vi "Merc_Connection_Check.vi"(0 "VISA resource name":refnum<visa-resource-name>="GPIB0::24::1::INSTR", 1 "IP Address":string, 5 "Comms Layer":T1=enum."GPIB", 7 "Serial Configuration":T3={"Baud Rate"=9600, "Parity"=0, "Data Bits"=8, "Stop Bits"=20, "Flow Control"=0} {"Flow Control" items=["None", "XON/XOFF", "RTS/CTS", "XON/XOFF & RTS/CTS", "DTR/DSR", "XON/XOFF & DTR/DSR"]; "Stop Bits" items=["1.0"=10, "2.0"=20]; "Data Bits" items=["7"=7, "8"=8]; "Parity" items=["None", "Odd", "Even"]; "Baud Rate" items=["300"=300, "600"=600, "1200"=1200, "2400"=2400, "4800"=4800, "9600"=9600, "19200"=19200]}, 9 "ID Query (True)":bool, 12 "Clear Previous Connections (False)":bool, 13 "ISOBUS address":T2=-1 caption="ISOBUS address (-1)") -> (3 "Installed Devices":string[](array[string]), 14 "Valid?":T4, 15 "error out":errorcluster)   [LabVIEW 2013]
uses:
  <instrlib>/Mercury iXX/Public/Controls/Comms Transport Layer.ctl
  <instrlib>/Mercury iXX/Public/Controls/Serial Settings.ctl
  <instrlib>/Mercury iXX/Public/Controls/ISOBus Address.ctl
  <instrlib>/Mercury iXX/Public/Controls/Is Valid LED.ctl
  <instrlib>/Mercury iXX/Public/Libraries/System/Open/Open System.vi
  <instrlib>/Mercury iXX/Public/Libraries/System/Read/Catalogue (Read).vi
  <instrlib>/Mercury iXX/Public/Libraries/System/Read/Date (Read).vi
  <instrlib>/Mercury iXX/Public/Libraries/System/Read/FVer (Read).vi
  <instrlib>/Mercury iXX/Public/Libraries/System/Read/Serial Number (Read).vi
  <instrlib>/Mercury iXX/Public/Libraries/System/Read/Time (Read).vi
  <instrlib>/Mercury iXX/Mercury iXX.lvlib
  <instrlib>/Mercury iXX/Public/Libraries/System.lvlib
panel:
  in  "stop":bool
  in  "Tab Control":enum32{"Connection", "Devices"}(tab)
  out "VISA Comms Layer Notes":string
  in  "Connect":bool
  out "Connected?":bool
  out "Firmware Version":string
  out "Main Board Serial Number":string
  out "Mercury Sys Date":string
  out "Mercury Sys Time":string
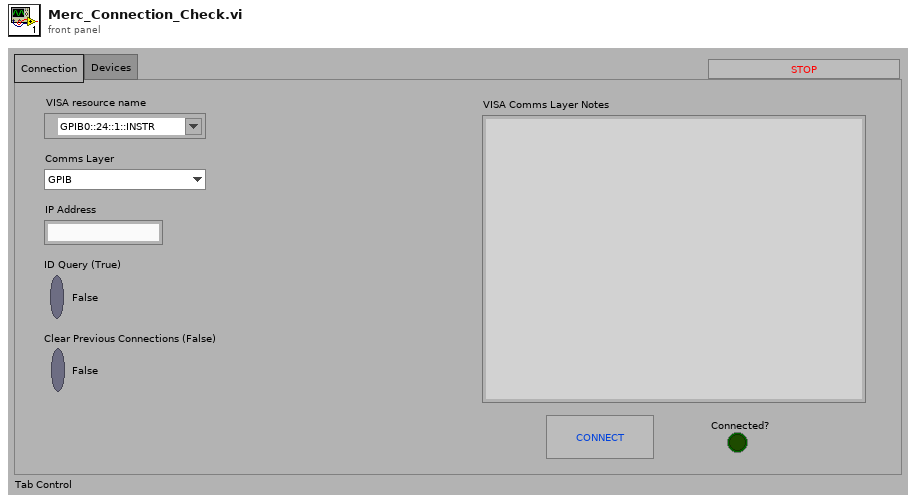
[diagram p1: front panel]
types:
  T1 = typedef "Mercury iXX.lvlib/Comms Transport Layer.ctl" = enum16{"Ethernet TCP/IP", "USB", "ISOBus - RS-232", "GPIB"}
  T2 = typedef "Mercury iXX.lvlib/ISOBus Address.ctl" = i32
  T3 = typedef "Mercury iXX.lvlib/Serial Settings.ctl" = cluster{"Baud Rate":u32, "Parity":u16, "Data Bits":u16, "Stop Bits":u16, "Flow Control":u16}
  T4 = typedef "Mercury iXX.lvlib/Is Valid LED.ctl" = bool
  T5 = typedef "Mercury iXX.lvlib/Mercury Reference.ctl" = cluster{"Comms":refnum<visa-resource-name>, "Device ID":string[], "Comms Layer":T1, "Command":string, "Query reference":T6}
  T6 = typedef "Mercury iXX.lvlib/Query Dynamic Reference.ctl" = refnum<vi>
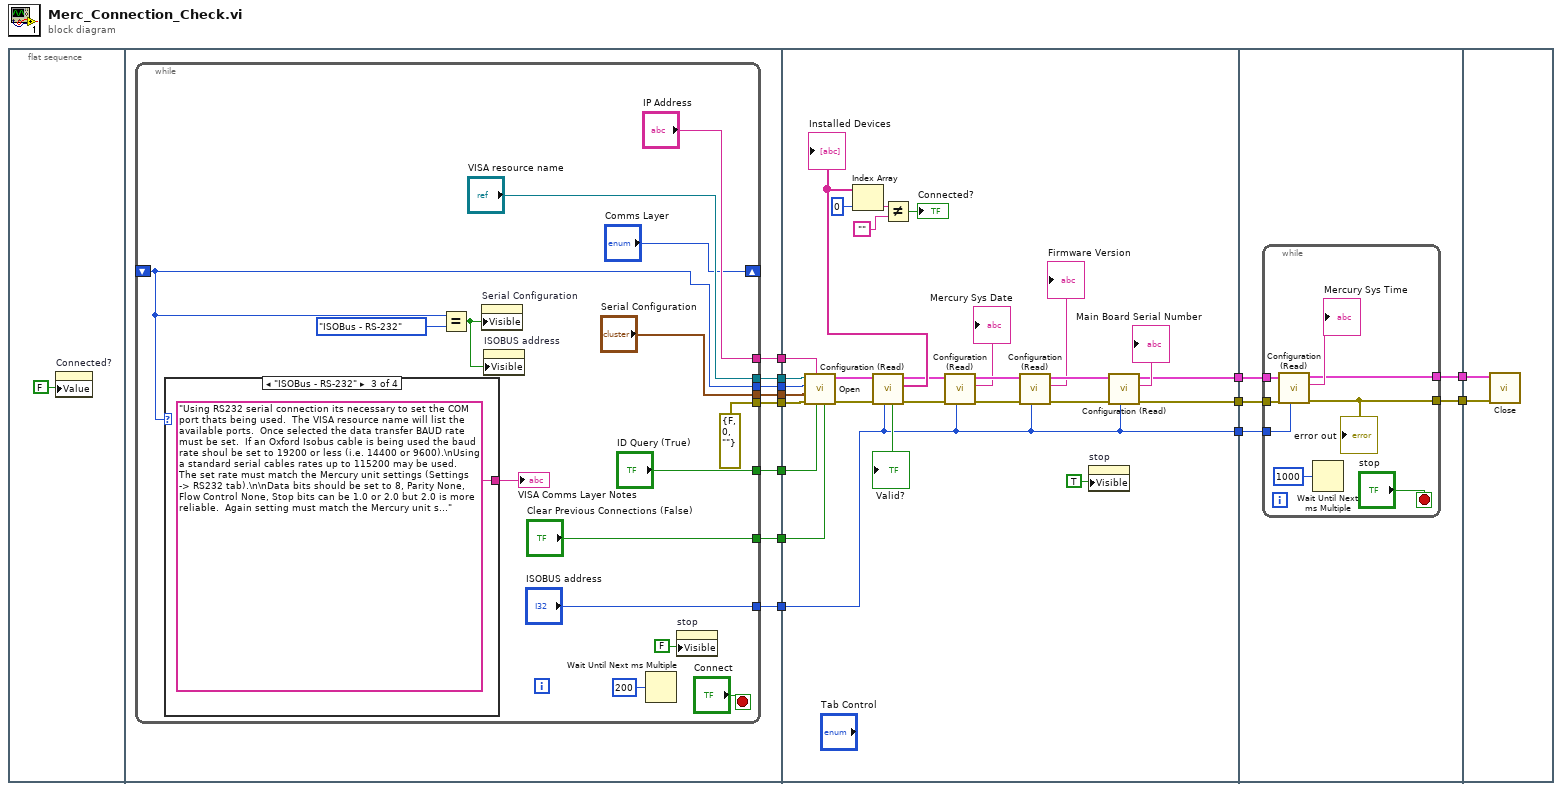
[diagram p0: block diagram]
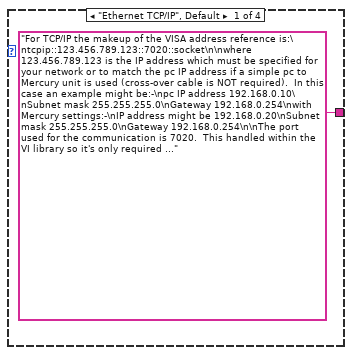
[diagram p2: hidden frame]
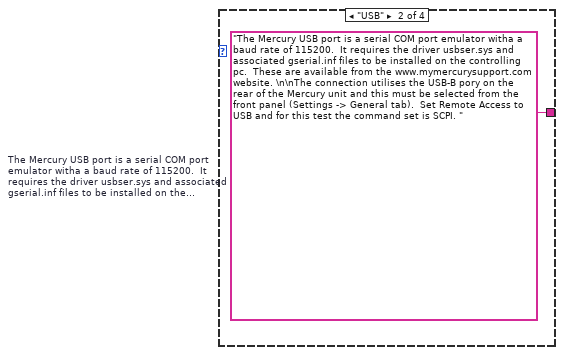
[diagram p3: hidden frame]
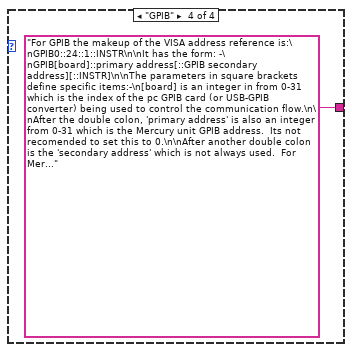
[diagram p4: hidden frame]
diagram:
  n1 = flat-sequence {
    tunnel: [w22] -> w13
    tunnel: [w21] -> w12
    tunnel: [w20] -> w11
    tunnel: [w19] -> w10
    tunnel: [w18] -> w9
    tunnel: [w17] -> w8
    tunnel: [w16] -> w7
    tunnel: [w15] -> w6
    tunnel: w13 -> [w64]
    tunnel: w12 -> [w63]
    tunnel: w11 -> [w65]
    tunnel: w10 -> [w66]
    tunnel: w9 -> [w67]
    tunnel: w8 -> [w69]
    tunnel: w7 -> [w68]
    tunnel: w6 -> [w43]
    tunnel: [w49] -> w5
    tunnel: [w43] -> w4
    tunnel: [w42] -> w3
    tunnel: w5 -> [w73]
    tunnel: w4 -> [w72]
    tunnel: w3 -> [w74]
    tunnel: [w71] -> w2
    tunnel: [w70] -> w1
    tunnel: w2 -> [w84]
    tunnel: w1 -> [w83]
    frame #0 {
      n2 = property on="Connected?" class="Bool (strict)"("Value"=FALSE ("x != y?")) -> ()  [unwired: 2 in, 2 out]
    }
    frame #1 {
      n3 = while {
        tunnel: ["VISA resource name"] -> w22
        tunnel: ["IP Address"] -> w21
        tunnel: [w25] -> w20
        tunnel: ["Serial Configuration"] -> w19
        tunnel: [errorcluster {"status"=FALSE, "code"=0, "source"=""} ("error in (no error)")] -> w18
        tunnel: ["ID Query (True)"] -> w17
        tunnel: ["Clear Previous Connections (False)"] -> w16
        tunnel: ["ISOBUS address"] -> w15
        shift-right: ["Comms Layer"] -> _
        shift-left: _ -> [w25]
        stop <- "Connect" stop-if-true
        n4 = case shown="\"ISOBus - RS-232\"" w25 {
          tunnel: ["For TCP/IP the makeup of the VISA address reference is:\ntcpip::123.456.789.123::7020::socket\n\nwhere 123.456.789.123 is the IP address which must be specified for your network or to match the pc IP address if a simple pc to Mercury unit is used (cross-over cable is NOT required).  In this case an example might be:-\npc IP address 192.168.0.10\nSubnet mask 255.255.255.0\nGateway 192.168.0.254\nwith Mercury settings:-\nIP address might be 192.168.0.20\nSubnet mask 255.255.255.0\nGateway 192.168.0.254\n\nThe port used for the communication is 7020.  This handled within the VI library so it's only required to set the IP address in the VI to Match the Mercury unit. \n\nTo use,TCP/IP must be selected from the Mercury front panel (Settings -> General tab).  Set Remote Access to Ethernet and for this test the command set is SCPI." w39 "Using RS232 serial connection its necessary to set the COM port thats being used.  The VISA resource name will list the available ports.  Once selected the data transfer BAUD rate must be set.  If an Oxford Isobus cable is being used the baud rate shoul be set to 19200 or less (i.e. 14400 or 9600).\nUsing a standard serial cables rates up to 115200 may be used.  The set rate must match the Mercury unit settings (Settings -> RS232 tab).\n\nData bits should be set to 8, Parity None, Flow Control None, Stop bits can be 1.0 or 2.0 but 2.0 is more reliable.  Again setting must match the Mercury unit settings.\n\nAlways set an Isobus address even if an Isobus cable is not used.  Some of the functions in the VI library expect an Isobus address when useing RS232 comms and will not respond if its missing.\n\nTo use, RS232 must be selected from the Mercury front panel (Settings -> General tab).  Set Remote Access to RS232 and for this test, the command set is SCPI." "For GPIB the makeup of the VISA address reference is:\nGPIB0::24::1::INSTR\n\nIt has the form: -\nGPIB[board]::primary address[::GPIB secondary address][::INSTR]\n\nThe parameters in square brackets define specific items:-\n[board] is an integer in from 0-31 which is the index of the pc GPIB card (or USB-GPIB converter) being used to control the communication flow.\n\nAfter the double colon, 'primary address' is also an integer from 0-31 which is the Mercury unit GPIB address.  Its not recomended to set this to 0.\n\nAfter another double colon is the 'secondary address' which is not always used.  For Mercury units it is used and set to 1.\n\nTo use, GPIB must be selected from the Mercury front panel (Settings -> General tab).  Set Remote Access to GPIB and for this test the command set is SCPI."] -> w28
          frame "Ethernet TCP/IP", Default {
          }
          frame "USB" {
            w39 = "The Mercury USB port is a serial COM port emulator witha a baud rate of 115200.  It requires the driver usbser.sys and associated gserial.inf files to be installed on the controlling pc.  These are available from the www.mymercurysupport.com website. \n\nThe connection utilises the USB-B pory on the rear of the Mercury unit and this must be selected from the front panel (Settings -> General tab).  Set Remote Access to USB and for this test the command set is SCPI. "  # The Mercury USB port is a serial COM port emulator witha a baud rate of 115200.  It requires the driver usbser.sys and associated gserial.inf files to be installed on the controlling pc.  These are available from the www.mymercurysupport.com website.   The connection utilises the USB-B pory on the rear of the Mercury unit and this must be selected from the front panel (Settings -> General tab).  Set Remote Access to USB and for this test the command set is SCPI.
          }
          frame "ISOBus - RS-232" {
          }
          frame "GPIB" {
          }
        }
        "VISA Comms Layer Notes" <- w28
        n5 = Equal?(x=w25, y=Comms_Transport_Layer."ISOBus - RS-232") -> (x = y?=w24:bool)
        n6 = property on="Serial Configuration" class="Clust (strict)"("Visible"=w24) -> ()  [unwired: 2 in, 2 out]
        n7 = property on="ISOBUS address" class="DigNum (strict)"("Visible"=w24) -> ()  [unwired: 2 in, 2 out]
        n8 = Wait Until Next ms Multiple(millisecond multiple=u32 200) -> ()  [unwired: 1 out]
        n9 = property on="stop" class="Bool"("Visible"=FALSE) -> ()  [unwired: 2 in, 2 out]
      }
    }
    frame #2 {
      n10 = call-poly <instrlib>:"Open.vi"("Clear Previous Connections (False)"=w68, "ID Query (True)"=w69, "IP Address"=w63, "error in (no error)"=w67, "Serial Configuration"=w66, "Comms Layer"=w65, "VISA resource name"=w64) -> ("error out"=w58:errorcluster, "Mercury Reference Out"=w59:T5)  [unwired: 3 out]
      n11 = call-poly <instrlib>:"Configuration (Read).vi"("ISOBUS address"=w43, "error in"=w58, "Mercury Reference In"=w59) -> ("error out"=w52:errorcluster, "Devices"=w56:string[], "Mercury Reference Out"=w53:T5, "Valid?"=→"Valid?":T4)  [unwired: 5 out]
      "Installed Devices" <- w56
      n12 = Index Array(array=w56, index=0) -> (element=w55:string)
      n13 = Not Equal?(x=w55, y="") -> (x != y?=→"Connected?":bool)
      n14 = call-poly <instrlib>:"Configuration (Read).vi"("ISOBUS address"=w43, "error in"=w52, "Mercury Reference In"=w53) -> ("error out"=w51:errorcluster, "Date"=→"Mercury Sys Date":string, "Mercury Reference Out"=w48:T5)  [unwired: 5 in, 1 out]
      n15 = call-poly <instrlib>:"Configuration (Read).vi"("ISOBUS address"=w43, "error in"=w51, "Mercury Reference In"=w48) -> ("error out"=w50:errorcluster, "Firmware Version"=→"Firmware Version":string, "Mercury Reference Out"=w47:T5)  [unwired: 5 in, 1 out]
      n16 = property on="stop" class="Bool"("Visible"=TRUE) -> ()  [unwired: 2 in, 2 out]
      n17 = call-poly <instrlib>:"Configuration (Read).vi"("ISOBUS address"=w43, "error in"=w50, "Mercury Reference In"=w47) -> ("error out"=w49:errorcluster, "Serial Number"=→"Main Board Serial Number":string, "Mercury Reference Out"=w42:T5)  [unwired: 5 in, 1 out]
    }
    frame #3 {
      n18 = while {
        tunnel: [w79] -> w71
        tunnel: [w78] -> w70
        tunnel: w74 -> [w77]
        tunnel: w73 -> [w76]
        tunnel: w72 -> [w75]
        stop <- "stop" stop-if-true
        n19 = call-poly <instrlib>:"Configuration (Read).vi"("ISOBUS address"=w75, "error in"=w76, "Mercury Reference In"=w77) -> ("error out"=w79:errorcluster, "Time"=→"Mercury Sys Time":string, "Mercury Reference Out"=w78:T5)  [unwired: 5 in, 1 out]
        "error out" <- w79
        n20 = Wait Until Next ms Multiple(millisecond multiple=u32 1000) -> ()  [unwired: 1 out]
      }
    }
    frame #4 {
      n21 = call <instrlib>:"Close.vi"("error in (no error)"=w84, "Mercury Reference"=w83) -> ()  [unwired: 9 in, 1 out]
    }
  }
